vi "Check Higher Warning.vi"(8 "error in (no error)":errorcluster, 10 "Input Values":sgl[](array[numeric]), 11 "AILimitConfig":T1(array[cluster])) -> (0 "error out":errorcluster, 3 "HW Channel":string[](array[string]))   [LabVIEW 2018]
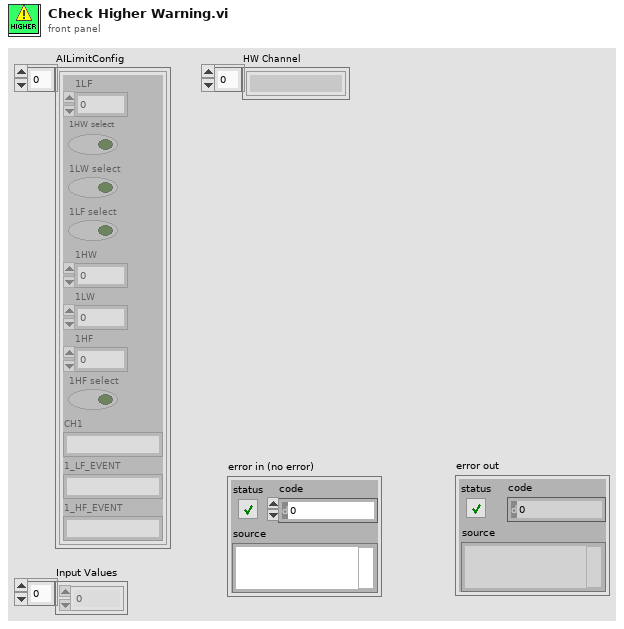
[diagram p1: front panel]
types:
  T1 = cluster{"1LF":dbl, "1HW select":bool, "1LW select":bool, "1LF select":bool, "1HW":dbl, "1LW":dbl, "1HF":dbl, "1HF select":bool, "CH1":string, "1_LF_EVENT":string, "1_HF_EVENT":string}[]
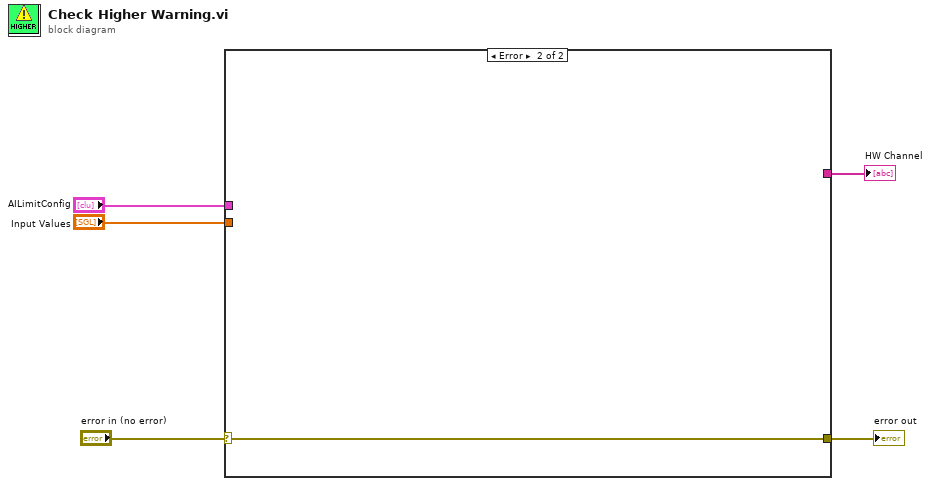
[diagram p0: block diagram]
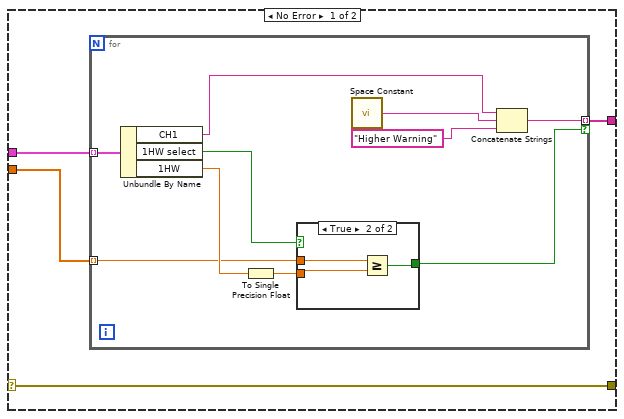
[diagram p2: hidden frame]
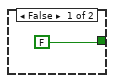
[diagram p3: hidden frame]
diagram:
  n1 = case shown="Error" "error in (no error)" {
    selector: "error in (no error)" -> [w6 w24]
    tunnel: "Input Values" -> [w9 _]
    tunnel: [w8 _] -> w4
    tunnel: "AILimitConfig" -> [w7 _]
    tunnel: [w6 w24] -> w1
    frame No Error {
      n2 = for {
        tunnel: w7 -> [w19] mode=indexing
        tunnel: w9 -> [w16] mode=indexing
        tunnel: [w12] -> w8 mode=indexing if=w11
        n3 = Unbundle By Name(w19) -> ("CH1"=w13:string, "1HW select"=w18:bool, "1HW"=w17:dbl)
        n4 = To Single Precision Float(number=w17) -> (single precision float=w10:sgl)
        n5 = case shown="True" w18 {
          tunnel: w16 -> [_ w23]
          tunnel: w10 -> [_ w22]
          tunnel: [FALSE w21] -> w11
          frame False {
          }
          frame True {
            n6 = Greater Or Equal?(x=w23, y=w22) -> (x >= y?=w21:bool)
          }
        }
        n7 = call <vilib>:"Space Constant.vi"() -> ("String"=w15:string)
        n8 = Concatenate Strings(w13, w15, "Higher Warning" ("string")) -> (w12:string)
      }
    }
    frame Error {
    }
  }
  "HW Channel" <- w4
  "error out" <- w1
